vi "Test Reference Channel Source.vi"(8 "error in (no error)":errorcluster, 11 "SR7270 Drivers in":refnum<class "SR7270 Drivers.lvclass">) -> (0 "error out":errorcluster, 3 "SR7270 Drivers out":refnum<class "SR7270 Drivers.lvclass">)   [LabVIEW 2016, in "SR7270 Drivers.lvlib"]
uses:
  SR7270 Drivers.lvlib
  <vilib>/addons/_JKI Toolkits/Caraya/classes/Assert/Assert.lvclass
  <vilib>/addons/_JKI Toolkits/Caraya/classes/Test/Test.lvclass
  Typedefs/IE--enum.ctl
  Typedefs/REFMODE--enum.ctl
  Typedefs/VRLOCK--enum.ctl
  SR7270 Drivers.lvclass
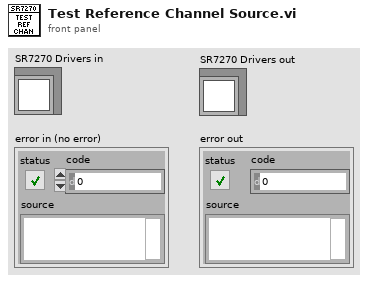
[diagram p1: front panel]
types:
  T1 = typedef "SR7270 Drivers.lvlib/VRLOCK--enum.ctl" = enum16{"Disabled", "Enabled"}
  T2 = typedef "SR7270 Drivers.lvlib/REFMODE--enum.ctl" = enum16{"Single Reference/Virtual Reference", "Dual Harmonic", "Dual Reference"}
  T3 = typedef "SR7270 Drivers.lvlib/IE--enum.ctl" = enum16{"Internal", "External (Rear Panel TTLREF IN)", "External (Front panel REF)"}
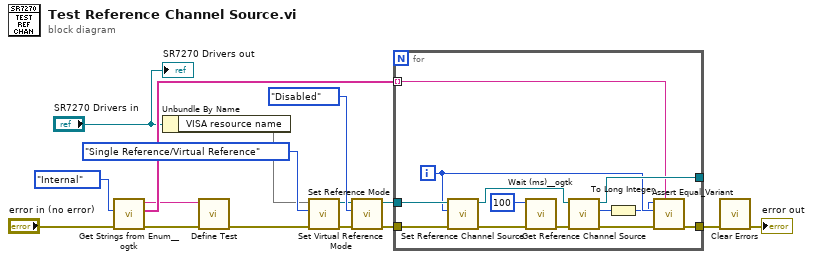
[diagram p0: block diagram]
diagram:
  n1 = call <userlib>:"Get Strings from Enum__ogtk.vi"("error in (no error)"="error in (no error)", "Enum"=IE--enum."Internal" ("Reference Channel")) -> ("error out"=w11:errorcluster, "Enum Strings"=w14:string[], "Enum Name"=w12:string)  [unwired: 6 in, 1 out]
  n2 = Unbundle By Name("SR7270 Drivers in") -> ("VISA resource name"=w2)
  n3 = call <vilib>:"Define Test.vi"("error in (no error)"=w11, "Label (VI Title)"=w12) -> ("error out"=w4:errorcluster)  [unwired: 9 in]
  n4 = call "Set Reference Mode.vi"("error in (no error)"=w4, "Reference Mode"=REFMODE--enum."Single Reference/Virtual Reference", "VISA resource name"=w2) -> ("error out"=w7:errorcluster, "VISA resource name out"=w6:refnum<visa-resource-name>)  [unwired: 7 in]
  n5 = call "Set Virtual Reference Mode.vi"("error in (no error)"=w7, "Virtual Reference Lock"=VRLOCK--enum."Disabled", "VISA resource name"=w6) -> ("error out"=w3:errorcluster, "VISA resource name out"=w5:refnum<visa-resource-name>)  [unwired: 7 in]
  n6 = for {
    tunnel: w5 -> [w28]
    tunnel: w3 -> [w20]
    tunnel: [w26] -> w16
    tunnel: [w25] -> _
    tunnel: w14 -> [w17] mode=indexing
    i -> [w19]
    n7 = call "Set Reference Channel Source.vi"("error in (no error)"=w20, "Reference Channel"=w19, "VISA resource name"=w28) -> ("error out"=w22:errorcluster, "VISA resource name out"=w29:refnum<visa-resource-name>)  [unwired: 7 in]
    n8 = call <userlib>:"Wait (ms)__ogtk.vi"("error in (no error)"=w22, "milliseconds to wait"=u32 100) -> ("error out"=w24:errorcluster)  [unwired: 8 in, 1 out]
    n9 = call "Get Reference Channel Source.vi"("error in (no error)"=w24, "VISA resource name"=w29) -> ("error out"=w27:errorcluster, "Reference Channel"=w21:T3, "VISA resource name out"=w25:refnum<visa-resource-name>)  [unwired: 7 in]
    n10 = To Long Integer(number=w21) -> (32bit integer=w18:i32)
    n11 = call <vilib>:"Assert Equal_Variant.vi"("Label"=w17, "error in (no error)"=w27, "Y"=w19, "X"=w18) -> ("error out"=w26:errorcluster)  [unwired: 7 in]
  }
  n12 = call <vilib>:"Clear Errors.vi"("error in (no error)"=w16) -> ("error out"=→"error out":errorcluster)  [unwired: 5 in, 1 out]
  "SR7270 Drivers out" <- "SR7270 Drivers in"
